vi "ActionVIOnCompile.vi"(8 "error in (no error)":errorcluster, 11 "Device Item Ref in":T1 format="%.0x") -> (0 "error out":errorcluster)   [LabVIEW 2015, in "Instrument Addon System Explorer.lvlib"]
uses:
  Instrument Addon System Explorer.lvlib
  <vilib>/NI Veristand/Custom Device API/Custom Device Item Ref.ctl
  Shared/Types/Compiled Settings.ctl
  Shared/Types/Command Parameters.ctl
  Shared/Types/Linked Channel Cluster.ctl
  Shared/Types/Response RT Configuration Cluster.ctl
  Shared/Types/Response Parameters.ctl
  Shared/Types/Response Wait Type.ctl
  Shared/Types/Message Parameters.ctl
  Shared/Types/Message Generation Type.ctl
  Shared/Types/External Trigger Refs.ctl
  <vilib>/NI Veristand/Custom Device API/Data Reference.ctl
  Types/Channel Lookup Cluster.ctl
  Types/Message Channel Lookup Cluster.ctl
  Shared/Types/FG Control.ctl
  Shared/Constants.vi
  <vilib>/NI Veristand/Custom Device API/NI VeriStand - Get Item Property.vi
  <vilib>/NI Veristand/Custom Device API/Get Item Property (U32).vi
  <vilib>/NI Veristand/Custom Device API/Set Item Property (U32).vi
  <vilib>/NI Veristand/Custom Device Tools/Custom Device Utility Library/NI VeriStand - Search for All Items by GUID.vi
  <vilib>/NI Veristand/Custom Device API/Get Item Property (Double).vi
  <vilib>/NI Veristand/Custom Device API/Get Item Property (Boolean).vi
  <vilib>/NI Veristand/Custom Device API/Get Item Property (String).vi
  <vilib>/NI Veristand/Custom Device API/Set Item Property (Double).vi
  <vilib>/NI Veristand/Custom Device API/Set Item Property (Boolean).vi
  <vilib>/NI Veristand/Custom Device API/Set Item Property (String).vi
  <vilib>/NI Veristand/Custom Device Tools/Custom Device Utility Library/NI VeriStand - Get Target Ref.vi
  <vilib>/NI Veristand/Custom Device API/NI VeriStand - Get Channel Data Reference.vi
  <vilib>/NI Veristand/Custom Device Tools/Custom Device Utility Library/NI VeriStand - Get Item Ref by Relative Path.vi
  <vilib>/NI Veristand/Custom Device API/Set Item Property (Variant).vi
  Shared/Instrument Addon Shared.lvlib
  <vilib>/NI VeriStand/Custom Device API/Custom Device API.lvlib
  <vilib>/NI Veristand/Custom Device Tools/Custom Device Utility Library/Custom Device Utility Library.lvlib
  <vilib>/NI/NI VeriStand Inline Async API/_Data Access System Explorer/Data Access System Explorer.lvlib
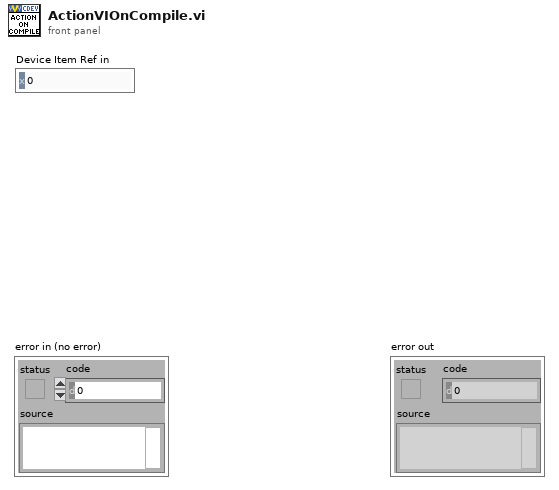
[diagram p1: front panel]
types:
  T1 = typedef "Custom Device API.lvlib/Custom Device Item Ref.ctl" = u64
  T2 = enum16{"Output/Write", "Input/Read", "Input/ReadWrite"}
  T3 = typedef "Instrument Addon Shared.lvlib/FG Control.ctl" = enum16{"Get", "Set"}
  T4 = typedef "Instrument Addon System Explorer.lvlib/Message Channel Lookup Cluster.ctl" = cluster{"Status":T1[], "Triggers":T1[], "Periodic Enable":T1[]}
  T5 = typedef "Instrument Addon Shared.lvlib/Compiled Settings.ctl" = cluster{"Command Parameters":T6[], "MetaData Lookup":variant, "Name":string, "Data Lookup":variant, "Response Parameters":T8[], "Message Generation Settings":T11[], "Wait Value Lookup":variant, "Decimation":u32, "External Channels":T13}
  T6 = typedef "Instrument Addon Shared.lvlib/Command Parameters.ctl" = cluster{"Command":string, "Linked Channels":T7[], "Pad":bool, "Length":u32, "Pad Value":u8}
  T7 = typedef "Instrument Addon Shared.lvlib/Linked Channel Cluster.ctl" = cluster{"Variable Name":string, "GUID":string}
  T8 = typedef "Instrument Addon Shared.lvlib/Response RT Configuration Cluster.ctl" = cluster{"Reponse Parameters":T9, "Use?":bool}
  T9 = typedef "Instrument Addon Shared.lvlib/Response Parameters.ctl" = cluster{"Response":string, "Linked Channels":T7[], "Type Value":dbl, "Wait Type":T10, "Use Channel":bool, "Channel Path":string}
  T10 = typedef "Instrument Addon Shared.lvlib/Response Wait Type.ctl" = enum16{"Byte Count", "Wait sec"}
  T11 = typedef "Instrument Addon Shared.lvlib/Message Parameters.ctl" = cluster{"Generation Type":T12, "Period":dbl, "Include Protection":bool, "Type":string}
  T12 = typedef "Instrument Addon Shared.lvlib/Message Generation Type.ctl" = enum16{"Trigger Only", "Periodic & Trigger"}
  T13 = typedef "Instrument Addon Shared.lvlib/External Trigger Refs.ctl" = cluster{"Channels":T14[], "Triggers":T14[], "Values":dbl[]}
  T14 = typedef "Custom Device API.lvlib/Data Reference.ctl" = i32
  T15 = cluster{"Name":string, "Type":enum16{"Output/Write", "Input/Read", "Input/ReadWrite"}, "VS Refs":T1[]}
  T16 = typedef "Instrument Addon System Explorer.lvlib/Channel Lookup Cluster.ctl" = cluster{"Lookup":variant, "Index":i32, "Refs":T1[]}
  T17 = typedef "Custom Device API.lvlib/Custom Device Item Info.ctl" = cluster{"Name":string, "Is Channel":bool, "GUID":string, "Is Waveform":bool}
  T18 = typedef "Instrument Addon Shared.lvlib/Trigger Parameters.ctl" = cluster{"Use Channel":bool, "Channel Path":string}
  T19 = cluster{"Name":string, "Type":enum16{"Output/Write", "Input/Read", "Input/ReadWrite"}, "VS Refs":T1[]}[]
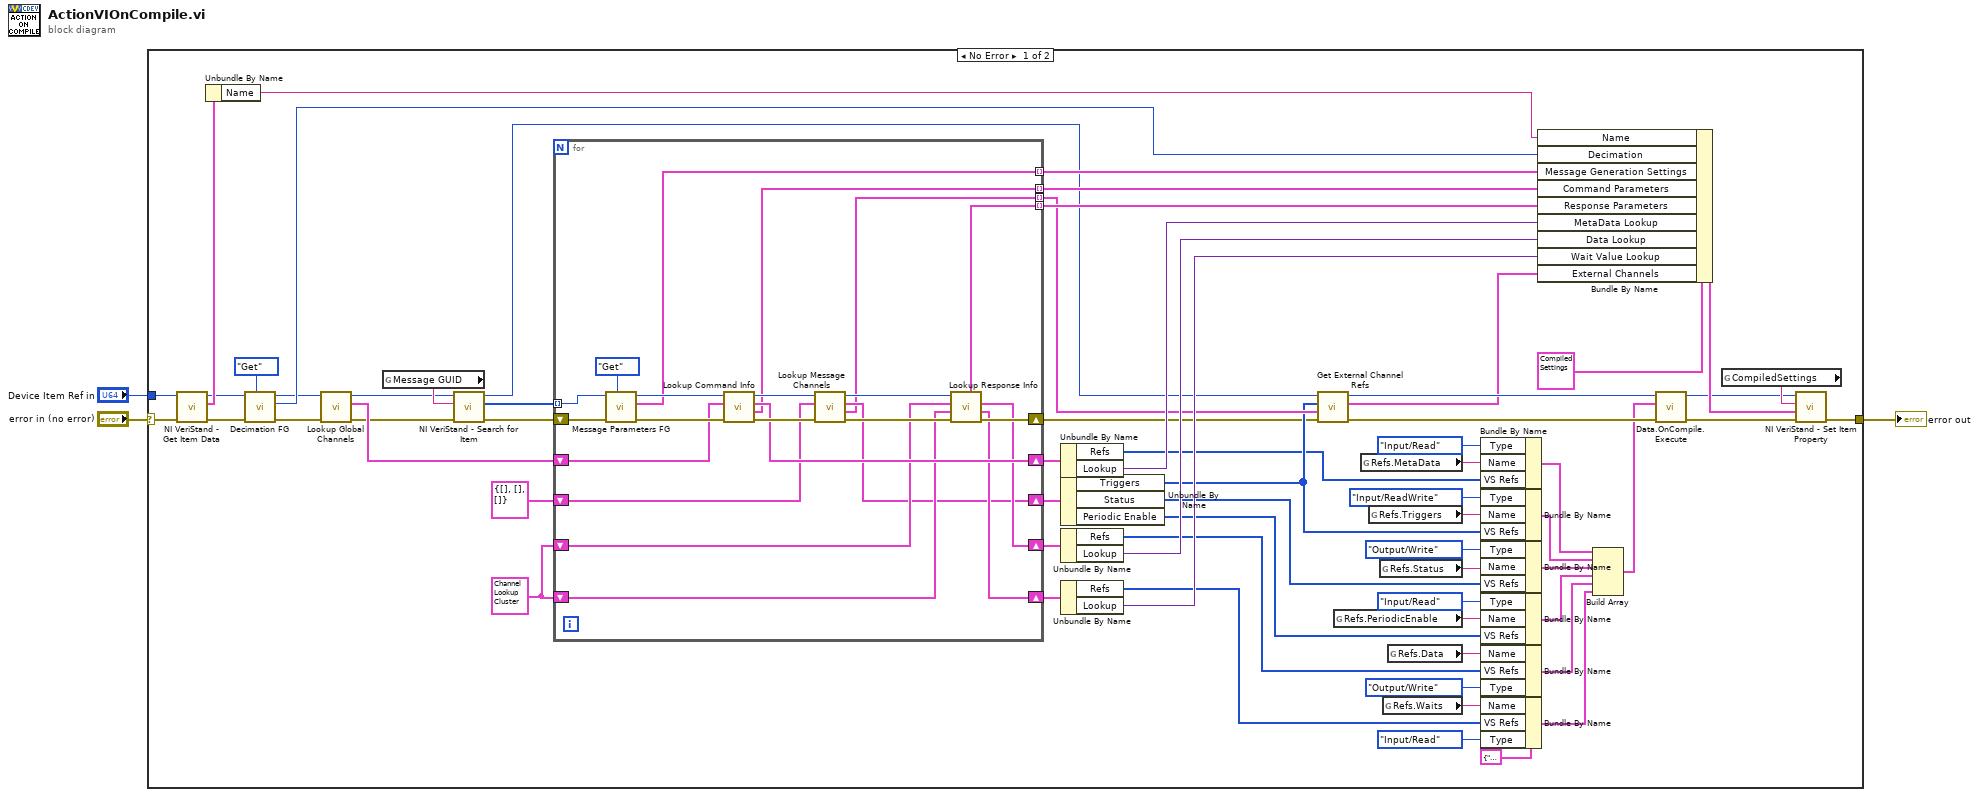
[diagram p0: block diagram]
diagram:
  n1 = case shown="No Error" "error in (no error)" {
    selector: "error in (no error)" -> [w44 w92]
    tunnel: [w43 w92] -> w2
    tunnel: "Device Item Ref in" -> [w45 _]
    frame No Error {
      w11 = T15 {"Name"="", "Type"=enum."Output/Write", "VS Refs"=[]} ("Group")
      w60 = T16 {"Lookup"=variant, "Index"=0, "Refs"=[]} ("Channel Lookup Info")
      n2 = call <vilib>:"NI VeriStand - Get Item Data.vi"("error in (no error)"=w44, "Item Ref in"=w45) -> ("error out"=w47:errorcluster, "Item Info"=w64:T17, "Item Ref out"=w48:T1)  [unwired: 6 in, 1 out]
      n3 = Unbundle By Name(w64) -> ("Name"=w9:string)
      n4 = call "Decimation FG.vi"("Action"=FG_Control."Get", "error in (no error)"=w47, "Device Item Ref in"=w48) -> ("error out"=w39:errorcluster, "Decimation out"=w50:u32, "Item Ref out"=w40:T1)  [unwired: 6 in]
      n5 = call "Lookup Global Channels.vi"("error in (no error)"=w39, "Item Ref in"=w40) -> ("error out"=w38:errorcluster, "Channel Lookup Info"=w61:T16, "Section Ref out"=w49:T1)  [unwired: 7 in]
      n6 = global read "Constants.vi" "Message GUID"() -> (w69:string)
      n7 = call-poly <vilib>:"NI VeriStand - Search for Item.vi"("error in"=w38, "Item GUID"=w69, "Section Ref in"=w49) -> ("error out"=w67:errorcluster, "Item Refs"=w68:T1[], "Section Ref out"=w30:T1)  [unwired: 5 in, 1 out]
      n8 = for {
        tunnel: w68 -> [w86] mode=indexing
        tunnel: [w72] -> w65 mode=indexing
        shift-right: [w89] -> w31
        shift-left: w67 -> [w88]
        tunnel: [w77] -> w63 mode=indexing
        tunnel: [w71] -> w62 mode=indexing
        shift-right: [w73] -> w54
        shift-left: T4 {"Status"=[], "Triggers"=[], "Periodic Enable"=[]} -> [w75]
        shift-right: [w82] -> w59
        shift-left: w61 -> [w83]
        shift-right: [w80] -> w57
        shift-left: w60 -> [w81]
        shift-right: [w79] -> w53
        shift-left: w60 -> [w78]
        tunnel: [w70] -> w46 mode=indexing
        n9 = call "Message Parameters FG.vi"("Action"=FG_Control."Get", "error in (no error)"=w88, "Item Ref in"=w86) -> ("error out"=w87:errorcluster, "Message Settings out"=w71:T11, "Item Ref out"=w85:T1)  [unwired: 6 in]
        n10 = call "Lookup Command Info.vi"("error in (no error)"=w87, "Channel Lookup Info in"=w83, "Item Ref in"=w85) -> ("error out"=w91:errorcluster, "Command Parameters"=w72:T6, "Channel Lookup Info out"=w82:T16, "Section Ref out"=w76:T1)  [unwired: 5 in]
        n11 = call "Lookup Message Channels.vi"("error in (no error)"=w91, "Message Channels in"=w75, "Section Ref in"=w76) -> ("error out"=w90:errorcluster, "Trigger Parameters"=w70:T18, "Message Channels out"=w73:T4, "Section Ref out"=w74:T1)  [unwired: 5 in]
        n12 = call "Lookup Response Info.vi"("error in (no error)"=w90, "Wait Value Channel Lookup Info"=w78, "Resp Channel Lookup Info"=w81, "Section Ref in"=w74) -> ("error out"=w89:errorcluster, "Wait Value Channel Lookup Info out"=w79:T16, "Resp Channel Lookup Info out"=w80:T16, "Response Info"=w77:T8)  [unwired: 3 in, 1 out]
      }
      n13 = Unbundle By Name(w59) -> ("Refs"=w8:T1[], "Lookup"=w58:variant)
      n14 = Unbundle By Name(w54) -> ("Triggers"=w32:T1[], "Status"=w7:T1[], "Periodic Enable"=w35:T1[])
      n15 = Unbundle By Name(w57) -> ("Refs"=w6:T1[], "Lookup"=w56:variant)
      n16 = Unbundle By Name(w53) -> ("Refs"=w5:T1[], "Lookup"=w52:variant)
      n17 = call "Get External Channel Refs.vi"("error in (no error)"=w31, "Triggers"=w46, "Internal Trigger Refs"=w32, "Device Ref in"=w30) -> ("error out"=w34:errorcluster, "Refs"=w4:T13, "Item Ref out"=w33:T1)  [unwired: 5 in]
      n18 = global read "Constants.vi" "Refs.PeriodicEnable"() -> (w27:string)
      n19 = global read "Constants.vi" "Refs.MetaData"() -> (w24:string)
      n20 = global read "Constants.vi" "Refs.Triggers"() -> (w25:string)
      n21 = global read "Constants.vi" "Refs.Status"() -> (w26:string)
      n22 = global read "Constants.vi" "Refs.Waits"() -> (w28:string)
      n23 = global read "Constants.vi" "Refs.Data"() -> (w29:string)
      n24 = Bundle By Name(cluster=w11, "Type"=T2."Input/Read", "Name"=w24, "VS Refs"=w8) -> (w17:T15)
      n25 = Bundle By Name(cluster=w11, "Type"=T2."Input/ReadWrite", "Name"=w25, "VS Refs"=w32) -> (w16:T15)
      n26 = Bundle By Name(cluster=w11, "Type"=T2."Output/Write", "Name"=w26, "VS Refs"=w7) -> (w15:T15)
      n27 = Bundle By Name(cluster=w11, "Type"=T2."Input/Read", "Name"=w27, "VS Refs"=w35) -> (w14:T15)
      n28 = Bundle By Name(cluster=w11, "Name"=w29, "VS Refs"=w6, "Type"=T2."Output/Write") -> (w13:T15)
      n29 = Bundle By Name(cluster=w11, "Name"=w28, "VS Refs"=w5, "Type"=T2."Input/Read") -> (w12:T15)
      n30 = Bundle By Name(cluster=T5 {"Command Parameters"=[], "MetaData Lookup"=variant, "Name"="", "Data Lookup"=variant, "Response Parameters"=[], "Message Generation Settings"=[], "Wait Value Lookup"=variant, "Decimation"=0, "External Channels"={"Channels"=[], "Triggers"=[], "Values"=[]}} ("Parameters"), "Name"=w9, "Decimation"=w50, "Message Generation Settings"=w62, "Command Parameters"=w65, "Response Parameters"=w63, "MetaData Lookup"=w58, "Data Lookup"=w56, "Wait Value Lookup"=w52, "External Channels"=w4) -> (w42:T5)
      n31 = Build Array(w17, w16, w15, w14, w13, w12) -> (w10:T19)
      n32 = call <vilib>:"Data.OnCompile.Execute.vi"("error in"=w34, "VS Ref Groups"=w10, "Custom Device Ref"=w33) -> ("error out"=w36:errorcluster, "Custom Device Ref"=w37:T1)  [unwired: 7 in]
      n33 = global read "Constants.vi" "CompiledSettings"() -> (w41:string)
      n34 = call-poly <vilib>:"NI VeriStand - Set Item Property.vi"("error in (no error)"=w36, "Value"=w42, "Property Name"=w41, "Item Ref in"=w37) -> ("error out"=w43:errorcluster)  [unwired: 5 in, 2 out]
    }
    frame Error {
    }
  }
  "error out" <- w2
